vi "GetHardwareLogColumnHeaders.vi"() -> (3 "Column Headers":string)   [LabVIEW 2012]
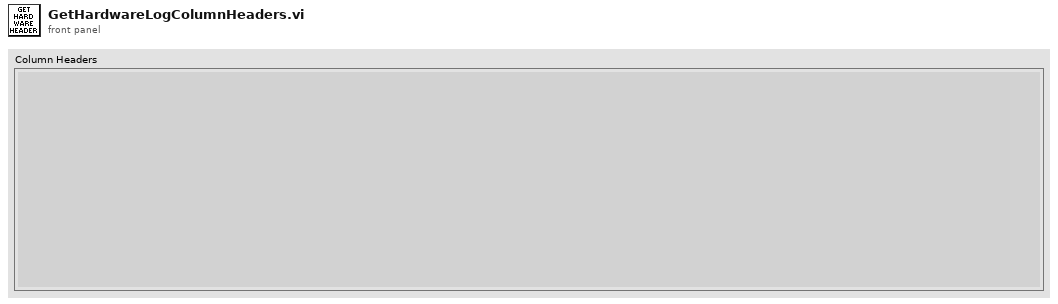
[diagram p1: front panel]
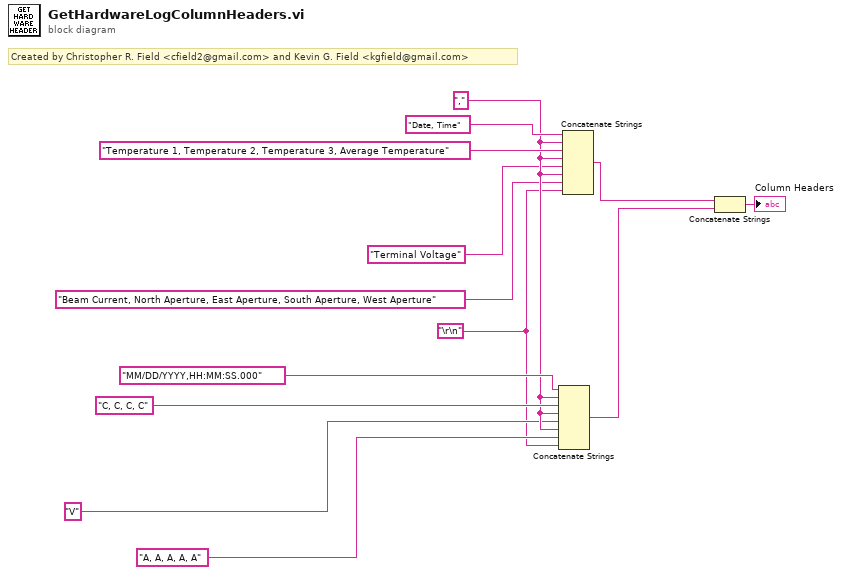
[diagram p0: block diagram]
diagram:
  w1 = "\r\n"
  w6 = ","
  # "Created by Christopher R. Field <cfield2@gmail.com> and Kevin G. Field <kgfield@gmail.com>"
  n1 = Concatenate Strings("MM/DD/YYYY,HH:MM:SS.000", w6, "C, C, C, C", w6, "V", w6, "A, A, A, A, A", w1) -> (w10:string)
  n2 = Concatenate Strings("Date, Time", w6, "Temperature 1, Temperature 2, Temperature 3, Average Temperature", w6, "Terminal Voltage", w6, "Beam Current, North Aperture, East Aperture, South Aperture, West Aperture", w1) -> (w11:string)
  n3 = Concatenate Strings(w11, w10) -> (→"Column Headers":string)
